vi "_Get Tools App Context.vi"(8 "error in":errorcluster) -> (0 "error out":errorcluster, 3 "Application Context":refnum<vi>)   [LabVIEW 2020, in "Panther Dasboard Scripting Hooks.lvlib"]
uses:
  Panther Dasboard Scripting Hooks.lvlib
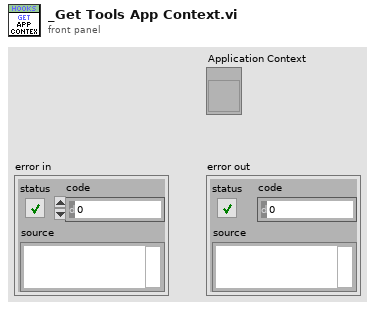
[diagram p1: front panel]
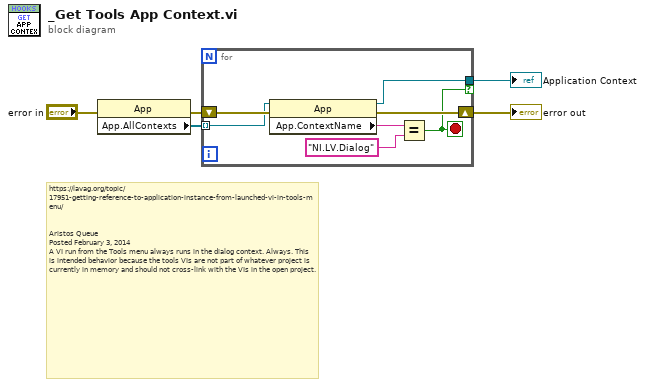
[diagram p0: block diagram]
diagram:
  # "https://lavag.org/topic/17951-getting-reference-to-application-instance-from-launched-vi-in-tools-menu/\n\n\nAristos Queue\nPosted February 3, 2014\nA VI run from the Tools menu always runs in the dialog context. Always. This is intended behavior because the tools VIs are not part of whatever project is currently in memory and should not cross-link with the VIs in the open project."
  n1 = property class="App"(error in="error in") -> (error out=w4:errorcluster, "App.AllContexts"=w2:refnum<vi>[])  [unwired: 1 in, 1 out]
  n2 = for {
    tunnel: w2 -> [w10] mode=indexing
    tunnel: [w7] -> w1 if=w6
    shift-right: [w11] -> w5
    shift-left: w4 -> [w12]
    stop <- w6 stop-if-true
    n3 = property class="App"(reference=w10, error in=w12) -> (reference out=w7:refnum<vi>, error out=w11:errorcluster, "App.ContextName"=w9:string)
    n4 = Equal?(x=w9, y="NI.LV.Dialog") -> (x = y?=w6:bool)
  }
  "Application Context" <- w1
  "error out" <- w5
